vi "change channel type.vi"(7 "owner ID":string, 8 "error in":errorcluster, 9 "new data type":T1, 10 "channel name":string, 11 "engine configuration in":refnum<class "base TBM sequencer configuration.lvclass">) -> (0 "error out":errorcluster, 3 "engine configuration out":refnum<class "base TBM sequencer configuration.lvclass">)   [LabVIEW 2014, in "base TBM sequencer configuration.lvclass"]
uses:
  base TBM sequencer configuration.lvclass
  <vilib>/NI/Tag Bus/tag/Data Type.ctl
  <vilib>/NI/Tag Bus/tag/tag descriptor.lvclass
  <vilib>/NI/Tag Bus/tag/tag descriptor.lvclass/tag descriptor.ctl
  base TBM sequencer configuration.lvclass/base TBM sequencer configuration.ctl
  <vilib>/NI/Tag Bus/tag/write data type.vi
  <vilib>/NI/Tag Bus/tag/write tag name.vi
  <vilib>/NI/Tag Bus Module Framework/channel/TBM channel.lvclass
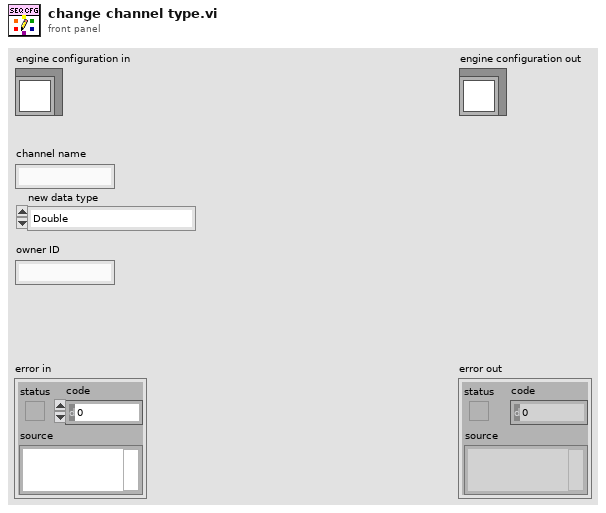
[diagram p1: front panel]
types:
  T1 = typedef "tag bus.lvlib/tag descriptor.lvclass/Data Type.ctl" = enum16{"Double", "Single", "I64", "I32", "I16", "I8", "U64", "U32", "U16", "U8", "Boolean", "String", "Array of Double", "Array of Single", "Array of I64", "Array of I32", "Array of I16", "Array of I8", "Array of U64", "Array of U32", "Array of U16", "Array of U8", "Array of Boolean", "Array of String"}
  T2 = typedef "base TBM sequencer configuration.lvclass/Tag Info.ctl" = cluster{"Channel":refnum<class "TBM channel.lvclass">, "Writers":string[], "Readers":string[], "Owning ID":string}
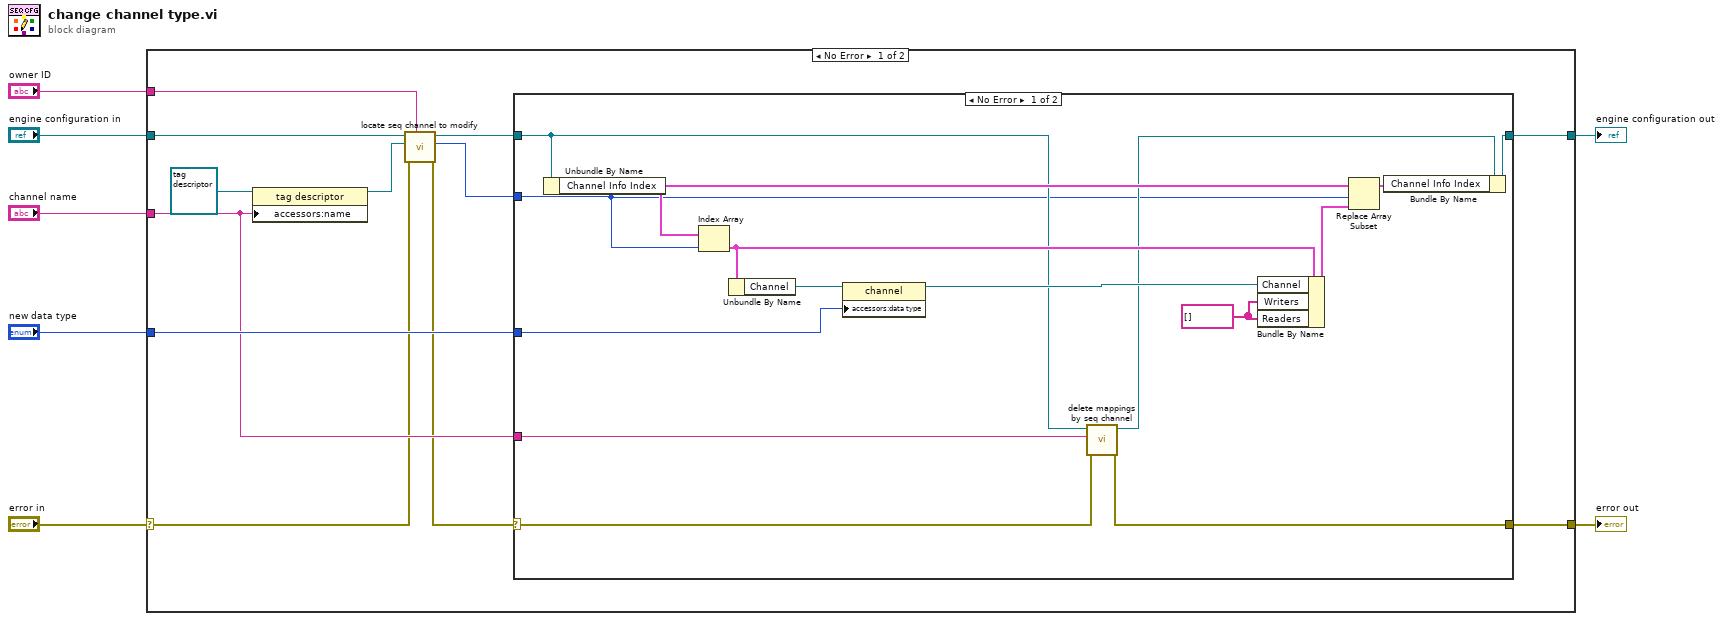
[diagram p0: block diagram]
diagram:
  n1 = case shown="No Error" "error in" {
    selector: "error in" -> [w10 w38]
    tunnel: [w17 w38] -> w6
    tunnel: [w18 w37] -> w4
    tunnel: "engine configuration in" -> [w14 w37]
    tunnel: "channel name" -> [w15 _]
    tunnel: "new data type" -> [w16 _]
    tunnel: "owner ID" -> [w11 _]
    frame No Error {
      n2 = property class="tag descriptor"(reference=refnum<class "tag descriptor.lvclass"> refnum ("tag descriptor"), "accessors:name"=w15) -> (reference out=w12:refnum<class "tag descriptor.lvclass">)  [unwired: 1 in, 1 out]
      n3 = call "locate seq channel to modify.vi"("owner ID"=w11, "error in"=w10, "tag descriptor"=w12, "engine configuration in"=w14) -> ("error out"=w9:errorcluster, "index"=w8:i32, "engine configuration out"=w13:refnum<class "base TBM sequencer configuration.lvclass">)  [unwired: 5 in]
      n4 = case shown="No Error" w9 {
        selector: w9 -> [w21 w35]
        tunnel: w13 -> [w26 w36]
        tunnel: [w27 w36] -> w18
        tunnel: [w25 w35] -> w17
        tunnel: w16 -> [w33 _]
        tunnel: w15 -> [w23 _]
        tunnel: w8 -> [w22 _]
        frame No Error {
          w20 = string[] [] ("Readers")
          n5 = Unbundle By Name(w26) -> ("Channel Info Index"=w30:T2[])
          n6 = Index Array(array=w30, index=w22) -> (element=w32:T2)
          n7 = Unbundle By Name(w32) -> ("Channel"=w34:refnum<class "TBM channel.lvclass">)
          n8 = property class="channel"(reference=w34, "accessors:data type"=w33) -> (reference out=w31:refnum<class "TBM channel.lvclass">)  [unwired: 1 in, 1 out]
          n9 = call "delete mappings by seq channel.vi"("error in"=w21, "seq channel name"=w23, "engine configuration in"=w26) -> ("error out"=w25:errorcluster, "engine configuration out"=w24:refnum<class "base TBM sequencer configuration.lvclass">)  [unwired: 7 in]
          n10 = Bundle By Name(cluster=w32, "Channel"=w31, "Writers"=w20, "Readers"=w20) -> (w29:T2)
          n11 = Replace Array Subset(array=w30, new element=w29, index=w22) -> (w28:T2[])
          n12 = Bundle By Name(cluster=w24, "Channel Info Index"=w28) -> (w27:refnum<class "base TBM sequencer configuration.lvclass">)
        }
        frame Error {
        }
      }
    }
    frame Error {
    }
  }
  "error out" <- w6
  "engine configuration out" <- w4
